vi "Time monitor.vi"(8 "error in (no error)":errorcluster, 11 "RxTx in":refnum<class "RxTx.lvclass">) -> (0 "error out":errorcluster, 3 "RxTx out":refnum<class "RxTx.lvclass">)   [LabVIEW 2018, in "RxTx.lvclass"]
uses:
  RxTx.lvclass
  RxTx.lvclass/RxTx.ctl
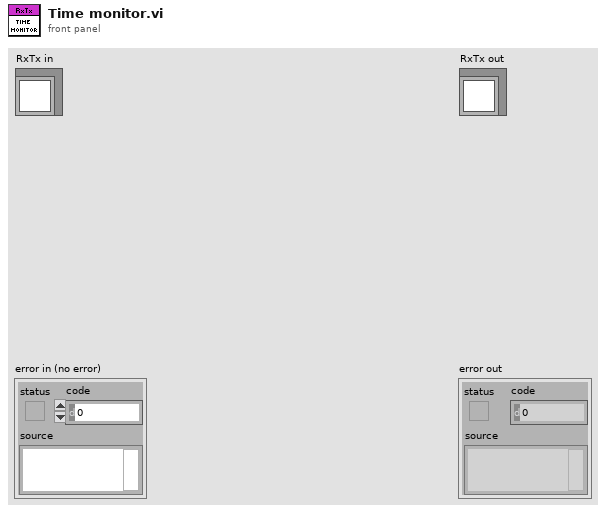
[diagram p1: front panel]
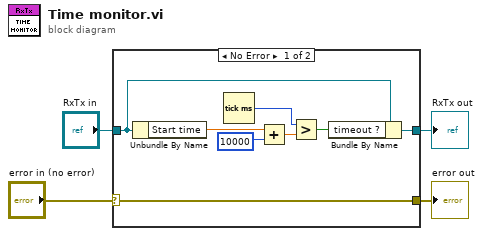
[diagram p0: block diagram]
diagram:
  n1 = case shown="No Error" "error in (no error)" {
    selector: "error in (no error)" -> [w12 w14]
    tunnel: [w12 w14] -> w3
    tunnel: [w11 w13] -> w1
    tunnel: "RxTx in" -> [w10 w13]
    frame No Error {
      n2 = Unbundle By Name(w10) -> ("Start time"=w7:dbl)
      n3 = Tick Count (ms)() -> (millisecond timer value=w9:u32)
      n4 = Add(x=w7, y=10000) -> (x+y=w5:dbl)
      n5 = Greater?(x=w9, y=w5) -> (0:w8:bool)
      n6 = Bundle By Name(cluster=w10, "timeout ?"=w8) -> (w11:refnum<class "RxTx.lvclass">)
    }
    frame Error {
    }
  }
  "error out" <- w3
  "RxTx out" <- w1
